vi "test.vi"() -> ()   [LabVIEW 2010]
uses:
  <vilib>/picture/picture.llb/Draw True-Color Pixmap.vi
  <vilib>/picture/3D Picture Control/NI_3D Picture Control.lvlib
panel:
  in  "Light Direction":dbl(knob)=314.8880943229338 scale=0.0..360.0 scale format="%.1f"
  in  "Style":bool=TRUE
  in  "Ratio":dbl=0.7 format="%.2f"
  in  "Colors":T1={"A Joint"=16711680, "A Span"=10066329, "B Joint"=255, "B Span"=16737843, "C Joint"=16711935, "C Claw"=39219}
  in  "Circle":T2={"top"=70.0, "left"=70.0, "height"=32.0, "width"=32.0} {"width" format="%.2f"; "height" format="%.2f"; "left" format="%.2f"; "top" format="%.2f"}
  out "Arm Picture":picture
  in  "Arm Parameters":T3={"Length A"=40.0, "Angle A"=0.0, "Length B"=30.0, "Angle B"=0.0, "Value Claw"=0.7, "Angle Claw"=0.0} {"Angle Claw" format="%.2f"; "Value Claw" format="%.2f"; "Angle B" format="%.2f"; "Length B" format="%.2f"; "Angle A" format="%.2f"; "Length A" format="%.2f"}
  in  "points":i32=180
  in  "start":dbl format="%0.2f"
  in  "increment":dbl=1.0 format="%0.2f"
  in  "polar attributes":T4={"maximum"=2.0, "minimum"=0.0, "clip to min"=FALSE, "log"=FALSE, "grid color"=3381657, "plot color"=16711680, "fmt and prec"={"format"=enum."Decimal", "precision"=2}, "visible section"=4} {"minimum" format="%0.2f"; "maximum" format="%0.2f"}
  in  "desired font":T5(ring)=enum."Application Font"
  out "?":picture
  in  "user-specified font":T6={"Font Name:"="monaco", "Size"=9, "Strikeout?"=FALSE, "Italic?"=FALSE, "Underline?"=FALSE, "Outline?"=FALSE, "Shadow?"=FALSE, "Bold?"=FALSE}
  out "3D Picture Control":refnum<vi>(3d-picture)
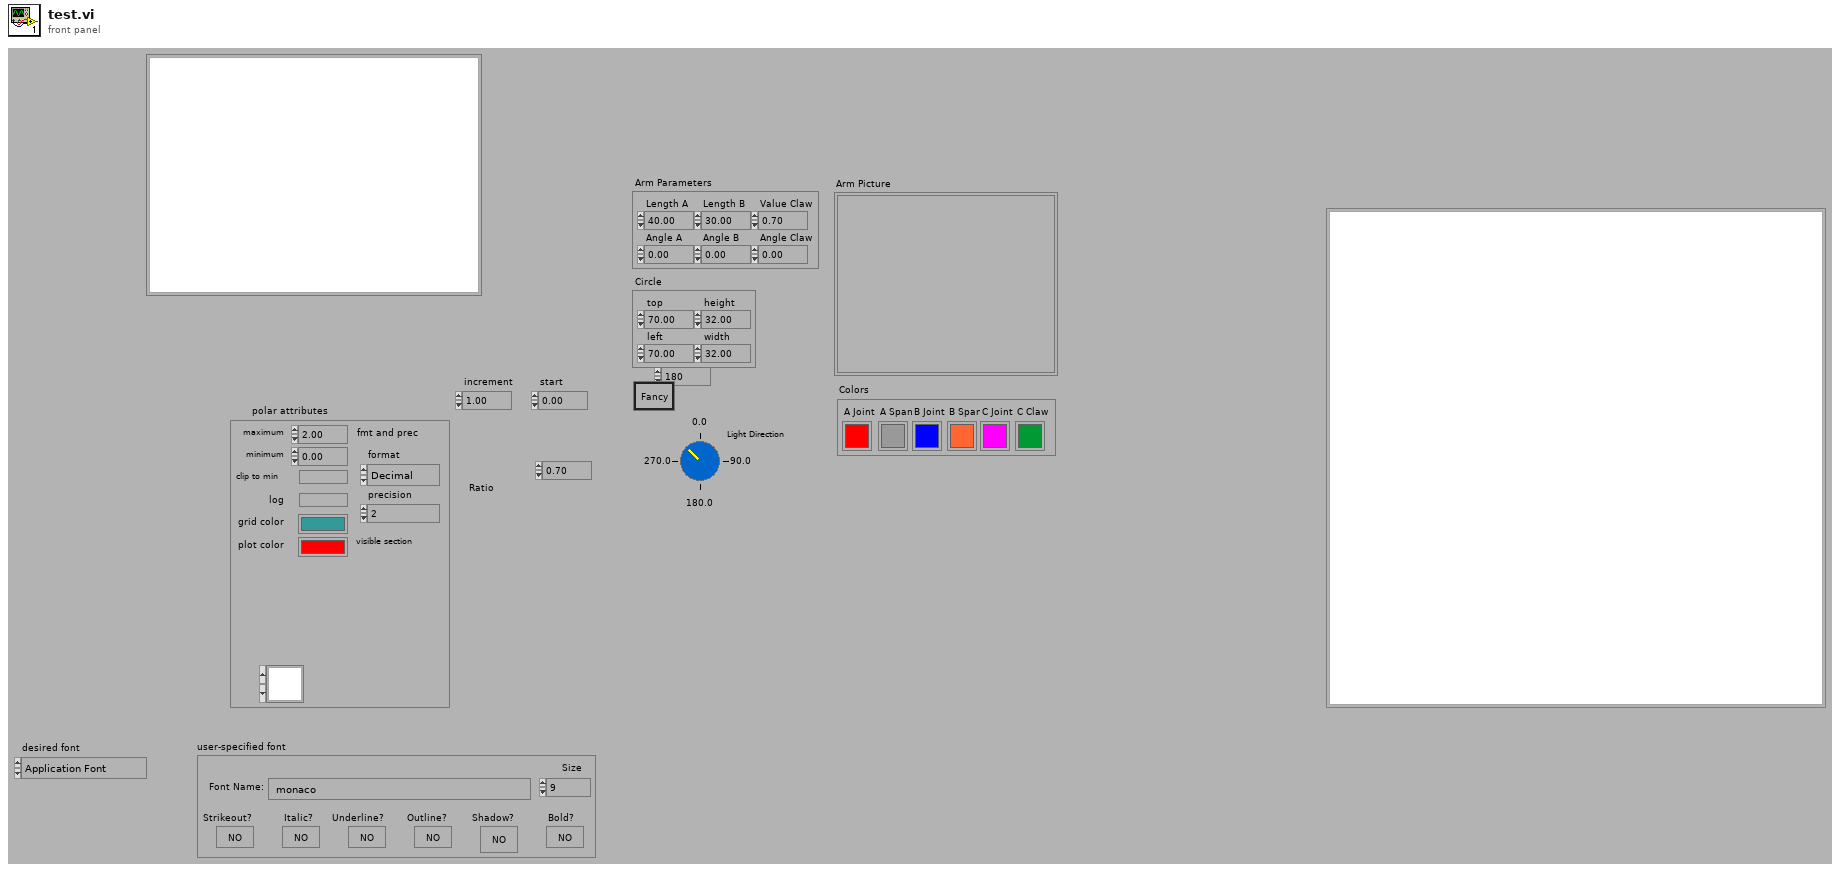
[diagram p1: front panel]
types:
  T1 = cluster{"A Joint":u32, "A Span":u32, "B Joint":u32, "B Span":u32, "C Joint":u32, "C Claw":u32}
  T2 = cluster{"top":dbl, "left":dbl, "height":dbl, "width":dbl}
  T3 = cluster{"Length A":dbl, "Angle A":dbl, "Length B":dbl, "Angle B":dbl, "Value Claw":dbl, "Angle Claw":dbl}
  T4 = cluster{"maximum":dbl, "minimum":dbl, "clip to min":bool, "log":bool, "grid color":u32, "plot color":u32, "fmt and prec":cluster{"format":enum8{"Decimal", "Scientific", "Engineering", "Binary", "Octal", "Hex"}, "precision":u8}, "visible section":u16}
  T5 = enum16{"User-specified Font", "Application Font", "System Font", "Dialog Font"}
  T6 = cluster{"Font Name:":string, "Size":i16, "Strikeout?":bool, "Italic?":bool, "Underline?":bool, "Outline?":bool, "Shadow?":bool, "Bold?":bool}
  T7 = enum16{"No Filtration", "Linear Filtration", "Simple Mipmap Filtration", "Bilinear Filtration", "Trilinear Filtration"}
  T8 = enum16{"As a Decal", "With Modulation", "With Blending", "As a replacement"}
  T9 = typedef "LVBoundsTypeDef.ctl" = cluster{"Width":u32, "Height":u32}
  T10 = typedef "imagedata.ctl" = cluster{"image type":i32, "image depth":i32, "image":u8[], "mask":u8[], "colors":u32[], "Rectangle":cluster{"left":i16, "top":i16, "right":i16, "bottom":i16}}
  T11 = cluster{"left":dbl, "top":dbl, "right":dbl, "bottom":dbl}
  T12 = cluster{"Angle A":dbl, "height":dbl, "Ratio":dbl}
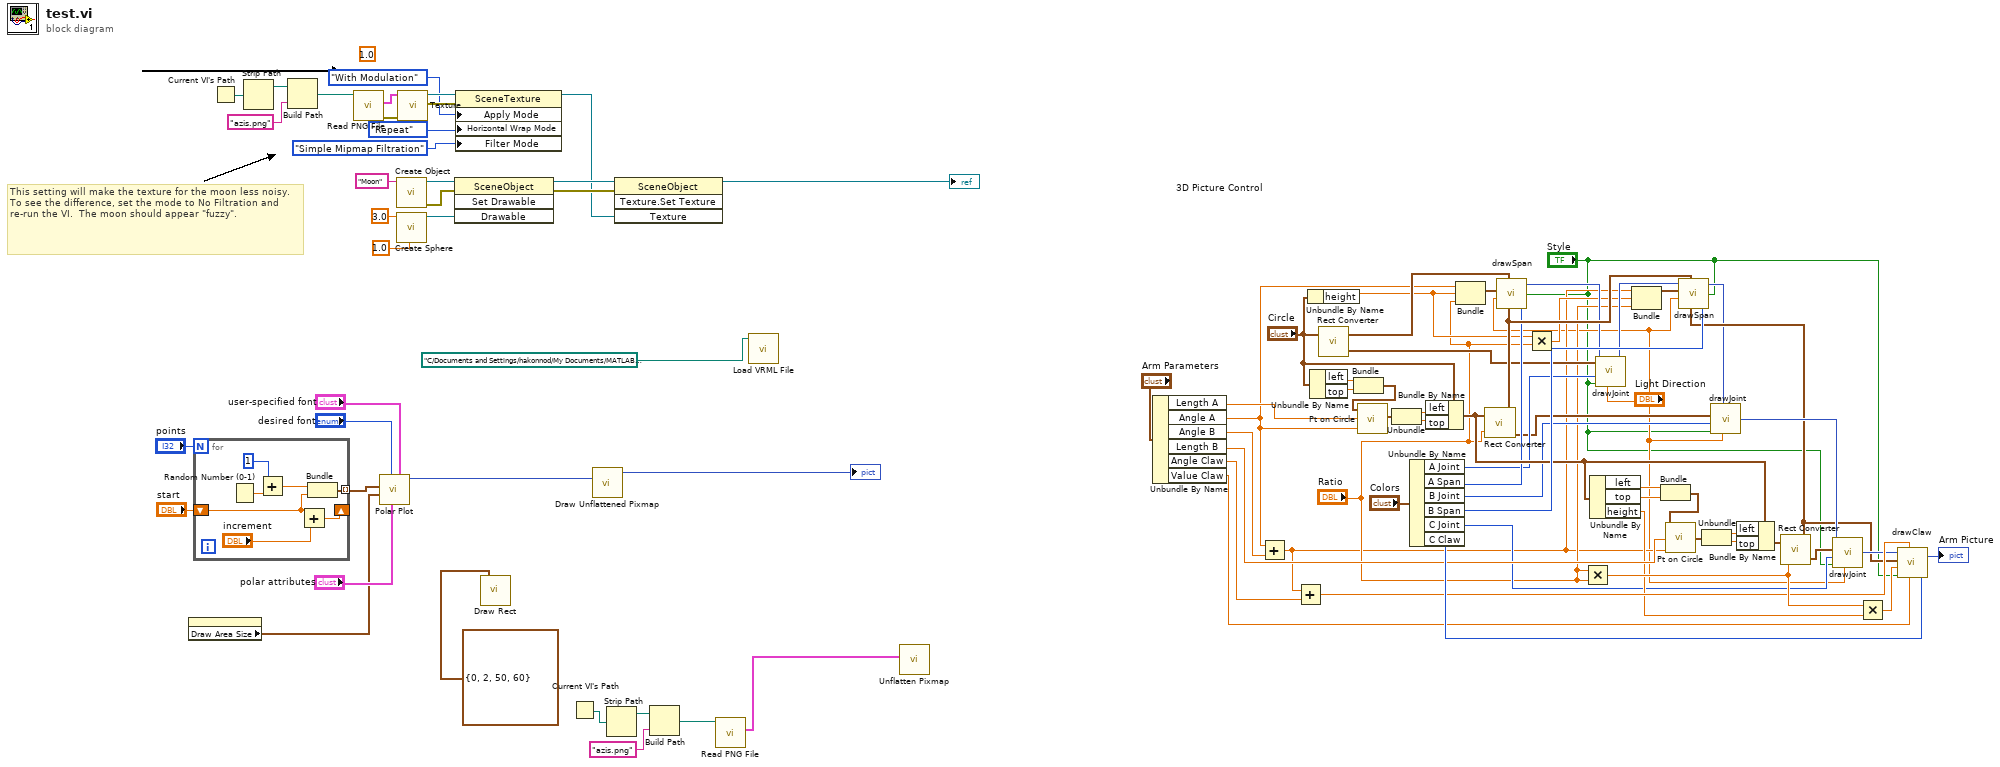
[diagram p0: block diagram]
diagram:
  (unwired) sgl 1.0 ("Detail")
  # "This setting will make the texture for the moon less noisy.\nTo see the difference, set the mode to No Filtration and\nre-run the VI.  The moon should appear \"fuzzy\"."
  n1 = property class="Pict"() -> ("Draw Area Size"=w63:T9)  [unwired: 2 in, 2 out]
  n2 = for {
    N: "points" -> [_]
    tunnel: [w97] -> w69 mode=indexing
    shift-right: [w95] -> _
    shift-left: "start" -> [w94]
    n3 = Random Number (0-1)() -> (number: 0 to 1=w92:dbl)
    n4 = Add(x=1, y=w92) -> (x+y=w91:dbl)
    n5 = Add(x=w94, y="increment") -> (x+y=w95:dbl)
    n6 = Bundle(w91, "start"=w94) -> (w97:cluster{dbl, "start":dbl})  [unwired: 1 in]
  }
  n7 = Current VI's Path() -> (path=w76:path)
  n8 = Strip Path(path=w76) -> (stripped path=w75:path)  [unwired: 1 out]
  n9 = Build Path(base path=w75, name or relative path="azis.png" ("Name")) -> (appended path=w73:path)
  n10 = call <vilib>:"Read PNG File.vi"("path to PNG file"=w73) -> ("error out"=w85:errorcluster, "image data"=w84:T10)  [unwired: 8 in, 1 out]
  n11 = call <vilib>:"Polar Plot.vi"("[user-specified font]"="user-specified font", "polar attributes"="polar attributes", "desired font(Application)"="desired font", "dimensions (w,h)"=w63, "data array [mag, phase (deg)]"=w69) -> ("new picture"=w4:picture)  [unwired: 6 in]
  n12 = call <vilib>:"Create Object.vi"("Name"="Moon") -> ("error out"=w87:errorcluster, "Scene:New Object"=w88:refnum<vi>)  [unwired: 1 in, 8 out]
  n13 = call <vilib>:"Create Sphere.vi"("Detail"=sgl 1.0, "Radius"=sgl 3.0) -> ("New Sphere Refnum"=w86:refnum<vi>)  [unwired: 1 in, 8 out]
  n14 = call <vilib>:"Texture.vi"("error in (no error)"=w85, "Image"=w84) -> ("error out"=w80:errorcluster, "New Texture Refnum"=w81:refnum<vi>)  [unwired: 8 out]
  n15 = invoke class="SceneObject" method="Set Drawable"(reference=w88, error in=w87, "Drawable"=w86) -> (reference out=w83:refnum<vi>, error out=w82:errorcluster)  [unwired: 1 in, 2 out]
  n16 = property class="SceneTexture"(reference=w81, error in=w80, "Apply Mode"=T8."With Modulation", "Horizontal Wrap Mode"=enum16{"Clamp", "Repeat"}."Repeat", "Filter Mode"=T7."Simple Mipmap Filtration") -> (reference out=w78:refnum<vi>)  [unwired: 1 out]
  n17 = call <vilib>:"Draw Rect.vi"("rect"=cluster{i32, i32, i32, i32} {0, 2, 50, 60}) -> ()  [unwired: 8 in, 1 out]
  n18 = Current VI's Path() -> (path=w61:path)
  n19 = call-poly <vilib>:"Draw Unflattened Pixmap.vi"("picture"=w4) -> ("new picture"=→"?":picture)  [unwired: 8 in]
  n20 = Strip Path(path=w61) -> (stripped path=w60:path)  [unwired: 1 out]
  n21 = invoke class="SceneObject" method="Texture.Set Texture"(reference=w83, error in=w82, "Texture"=w78) -> (reference out=→"3D Picture Control":refnum<vi>)  [unwired: 1 in, 3 out]
  n22 = Build Path(base path=w60, name or relative path="azis.png" ("Name")) -> (appended path=w58:path)
  n23 = call <vilib>:"Read PNG File.vi"("path to PNG file"=w58) -> ("image data"=w3:T10)  [unwired: 8 in, 2 out]
  n24 = call <vilib>:"Load VRML File.vi"("Path"=path "C:/Documents and Settings/hakonnod/My Documents/MATLAB/manualThrusterControl/boat/boat.wrl") -> ()  [unwired: 9 in, 2 out]
  n25 = call <vilib>:"Unflatten Pixmap.vi"("image data"=w3) -> ()  [unwired: 4 in, 7 out]
  n26 = Unbundle By Name("Arm Parameters") -> ("Length A"=w36:dbl, "Angle A"=w14:dbl, "Angle B"=w45:dbl, "Length B"=w26:dbl, "Angle Claw"=w44:dbl, "Value Claw"=w40:dbl)
  n27 = Add(x=w14, y=w45) -> (x+y=w9:dbl)
  n28 = Add(x=w9, y=w44) -> (x+y=w39:dbl)
  n29 = Unbundle By Name("Circle") -> ("height"=w15:dbl)
  n30 = Unbundle By Name("Circle") -> ("left"=w35:dbl, "top"=w34:dbl)
  n31 = call "Rect Converter.vi"("Rect"="Circle") -> ("Pict Rect"=w24:T11, "Center Pt"=w53:cluster{"X":dbl, "Y":dbl})  [unwired: 1 in]
  n32 = Bundle("left"=w35, "top"=w34) -> (w6:cluster{"left":dbl, "top":dbl})  [unwired: 1 in]
  n33 = call "Pt on Circle"("Angle"=w14, "Radius"=w36, "Center"=w6) -> ("Tangent Pt"=w33:cluster{"X":dbl, "Y":dbl})
  n34 = Unbundle(w33) -> ("X"=w32:dbl, "Y"=w31:dbl)
  n35 = Unbundle By Name("Colors") -> ("A Joint"=w23:u32, "A Span"=w46:u32, "B Joint"=w22:u32, "B Span"=w50:u32, "C Joint"=w20:u32, "C Claw"=w57:u32)
  n36 = Bundle By Name(cluster="Circle", "left"=w32, "top"=w31) -> (w47:T2)
  n37 = Bundle("Angle A"=w14, "height"=w15, "Ratio"="Ratio") -> (w13:T12)  [unwired: 1 in]
  n38 = call "Rect Converter.vi"("Scale Factor"="Ratio", "Rect"=w47) -> ("Pict Rect"=w21:T11, "Center Pt"=w48:cluster{"X":dbl, "Y":dbl})
  n39 = call "drawSpan.vi"("Center 1"=w53, "Circle Spec"=w13, "Light Direction"="Light Direction", "Center 2"=w48, "Style"="Style", "Color"=w46) -> ("Picture Out"=w18:picture)  [unwired: 2 in]
  n40 = Multiply(x=w15, y="Ratio") -> (x*y=w10:dbl)
  n41 = Multiply(x="Ratio", y="Ratio") -> (x*y=w42:dbl)
  n42 = Unbundle By Name(w47) -> ("left"=w30:dbl, "top"=w52:dbl, "height"=w25:dbl)
  n43 = call "drawJoint.vi"("Light Direction"="Light Direction", "Style"="Style", "Color"=w23, "Rectangle"=w24, "Picture In"=w18) -> ("Picture Out"=w17:picture)  [unwired: 1 in]
  n44 = Bundle(w9, w10, "Ratio"="Ratio") -> (w12:cluster{dbl, dbl, "Ratio":dbl})  [unwired: 1 in]
  n45 = Bundle("left"=w30, "top"=w52) -> (w8:cluster{"left":dbl, "top":dbl})  [unwired: 1 in]
  n46 = call "Pt on Circle"("Angle"=w9, "Radius"=w26, "Center"=w8) -> ("Tangent Pt"=w29:cluster{"X":dbl, "Y":dbl})
  n47 = Unbundle(w29) -> ("X"=w28:dbl, "Y"=w27:dbl)
  n48 = Bundle By Name(cluster=w47, "left"=w28, "top"=w27) -> (w51:T2)
  n49 = call "Rect Converter.vi"("Scale Factor"=w42, "Rect"=w51) -> ("Pict Rect"=w19:T11, "Center Pt"=w37:cluster{"X":dbl, "Y":dbl})
  n50 = call "drawSpan.vi"("Picture In"=w17, "Center 1"=w48, "Circle Spec"=w12, "Light Direction"="Light Direction", "Center 2"=w37, "Style"="Style", "Color"=w50) -> ("Picture Out"=w16:picture)  [unwired: 1 in]
  n51 = call "drawJoint.vi"("Light Direction"="Light Direction", "Style"="Style", "Color"=w22, "Rectangle"=w21, "Picture In"=w16) -> ("Picture Out"=w49:picture)  [unwired: 1 in]
  n52 = call "drawJoint.vi"("Light Direction"="Light Direction", "Style"="Style", "Color"=w20, "Rectangle"=w19, "Picture In"=w49) -> ("Picture Out"=w38:picture)  [unwired: 1 in]
  n53 = Multiply(x=w42, y=w25) -> (x*y=w41:dbl)
  n54 = call "drawClaw.vi"("Claw Color"=w57, "Claw Value"=w40, "Claw Angle"=w39, "Style"="Style", "Diameter"=w41, "Center"=w37, "Picture In"=w38) -> ("Picture Out"=→"Arm Picture":picture)
